vi "NI32LV110ASD8_Dashboard Main 3.vi"() -> ()   [LabVIEW 2011]
uses:
  <vilib>/Rock Robotics/WPI/DriverStation/WPI_DriverStationDigitalData.ctl
  3061 - Robot Code(Bob's)/Dashboard Datatype.ctl
panel:
  in  "Reset":bool
  out "Odometer":dbl
  out "Encoder Odometers":cluster{"Left Encoder":dbl, "Right Encoder":dbl}
  out "Launcher Rate":dbl(slide) scale=0.0..8.0
  out "Image Error Message":string
  in  "Viewer":enum32{"Camera Image", "Kinect Skeleton"}(tab)
  in  "Video Enable":bool
  out "Camera Image":T1(plugin-control)
  out "Buttons 1":cluster{"1":bool, "2":bool, "3":bool}
  out "Kinect 1":cluster{"X":dbl, "Y":dbl, "Z":dbl} {"X" scale=1.0..-1.0; "Y" scale=1.0..-1.0; "Z" scale=1.0..-1.0}
  out "Buttons 2":cluster{"1":bool, "2":bool, "3":bool}
  out "Kinect 2":cluster{"X":dbl, "Y":dbl, "Z":dbl} {"X" scale=1.0..-1.0; "Y" scale=1.0..-1.0; "Z" scale=1.0..-1.0}
  out "Version":string
  out "Skeleton Picture":picture
  out "Players":i8
  out "Robot IP Address":string
  out "Solenoid Output":bool[](array[boolean])
  out "Analog Input":sgl[](array[slide]) scale=0.0..5.0
  out "Relay":cluster{"Forward":bool[], "Reverse":bool[]}
  out "PWM":cluster{u8, u8}[](array[slide]) scale=1.0..255.0
  out "GPIO State":bool[](array[boolean])
  out "GPIO Output Enable":bool[](array[boolean])
  out "8 -- Battery":sgl(graph)
  out "Gyro":cluster{"Robot Gyro":dbl, "Robot Gyro":dbl}(knob) scale=-180.0..180.0
  out "Dashboard Datatype Warning":string
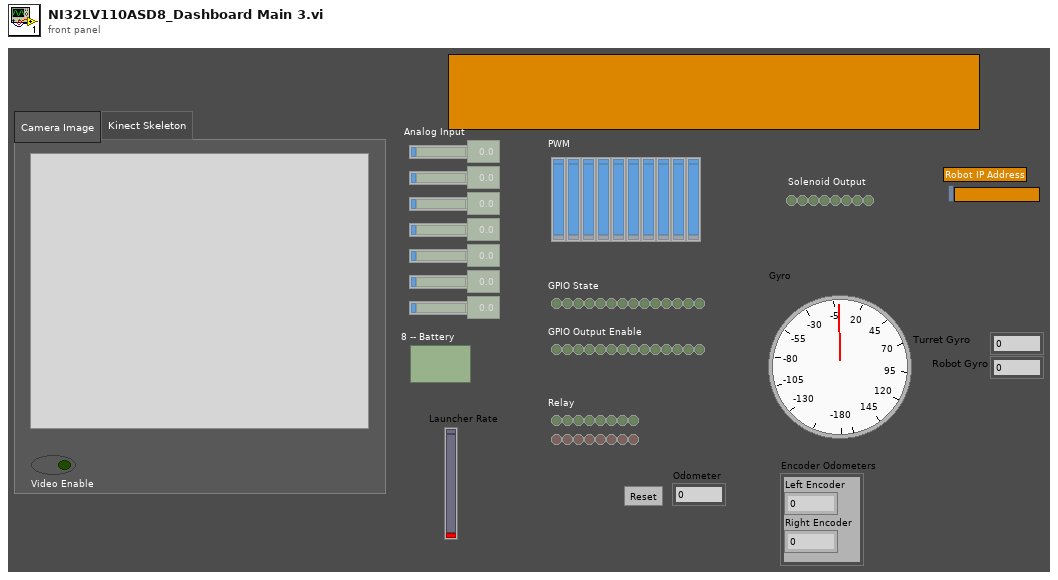
[diagram p1: front panel]
types:
  T1 = typedef "IMAQ Image.ctl" = refnum<image>
  T2 = typedef "Dashboard Datatype.ctl" = cluster{cluster{"AnalogModule[0]":cluster{"Channel[0]":sgl, "Channel[1]":sgl, "Channel[2]":sgl, "Channel[3]":sgl, "Channel[4]":sgl, "Channel[5]":sgl, "Channel[6]":sgl, "Channel[7]":sgl}, "AnalogModule[1]":cluster{"Channel[0]":sgl, "Channel[1]":sgl, "Channel[2]":sgl, "Channel[3]":sgl, "Channel[4]":sgl, "Channel[5]":sgl, "Channel[6]":sgl, "Channel[7]":sgl}}, cluster{"DigitalModule[0]":T3, "DigitalModule[1]":T3}, "Solenoid":u8, "Gyro":dbl, "Wheel Speed":dbl, "Arm Angle":dbl, "Arm Height":dbl, "Rack & Height":string}
  T3 = typedef "WPI_DriverStationDigitalData.ctl" = cluster{"Relay Fwd":u8, "Relay Rev":u8, "GPIO":u16, "GPIO_OE":u16, "PWM":cluster{"PWM[0]":u8, "PWM[1]":u8, "PWM[2]":u8, "PWM[3]":u8, "PWM[4]":u8, "PWM[5]":u8, "PWM[6]":u8, "PWM[7]":u8, "PWM[8]":u8, "PWM[9]":u8}}
  T4 = typedef "Image Type" = u32
  T5 = cluster{"Competition mode":bool, "Robot Link":bool, "Autonomous":bool, "Enabled":bool, "E-Stop":bool}
  T6 = cluster{"AnalogModule[0]":cluster{"Channel[0]":sgl, "Channel[1]":sgl, "Channel[2]":sgl, "Channel[3]":sgl, "Channel[4]":sgl, "Channel[5]":sgl, "Channel[6]":sgl, "Channel[7]":sgl}, "AnalogModule[1]":cluster{"Channel[0]":sgl, "Channel[1]":sgl, "Channel[2]":sgl, "Channel[3]":sgl, "Channel[4]":sgl, "Channel[5]":sgl, "Channel[6]":sgl, "Channel[7]":sgl}}
  T7 = cluster{"DigitalModule[0]":T3, "DigitalModule[1]":T3}
  T8 = cluster{"Channel[0]":sgl, "Channel[1]":sgl, "Channel[2]":sgl, "Channel[3]":sgl, "Channel[4]":sgl, "Channel[5]":sgl, "Channel[6]":sgl, "Channel[7]":sgl}[]
  T9 = cluster{"Channel[0]":sgl, "Channel[1]":sgl, "Channel[2]":sgl, "Channel[3]":sgl, "Channel[4]":sgl, "Channel[5]":sgl, "Channel[6]":sgl, "Channel[7]":sgl}
  T10 = typedef "LVRectTypeDef.ctl" = cluster{"left":i16, "top":i16, "right":i16, "bottom":i16}
  T11 = typedef "SkeletonTrackState.ctl" = enum32{"NotTracked", "PositionOnly", "Tracked"}
  T12 = cluster{"TrackingState":u8[], "Position":cluster{"x":sgl, "y":sgl, "z":sgl}, cluster{"x":sgl, "y":sgl, "z":sgl, sgl}[], "TrackState":T11}
  T13 = cluster{cluster{"ScaledToPercentRange":dbl, "ScaledToPercentRange":dbl, "ScaledToPercentRange":dbl}, cluster{bool, bool, bool}}[]
  T14 = typedef "LVBoundsTypeDef.ctl" = cluster{"Width":u32, "Height":u32}
  T15 = cluster{cluster{"ScaledToPercentRange":dbl, "ScaledToPercentRange":dbl, "ScaledToPercentRange":dbl}, cluster{bool, bool, bool}}
  T16 = cluster{"ScaledToPercentRange":dbl, "ScaledToPercentRange":dbl, "ScaledToPercentRange":dbl}
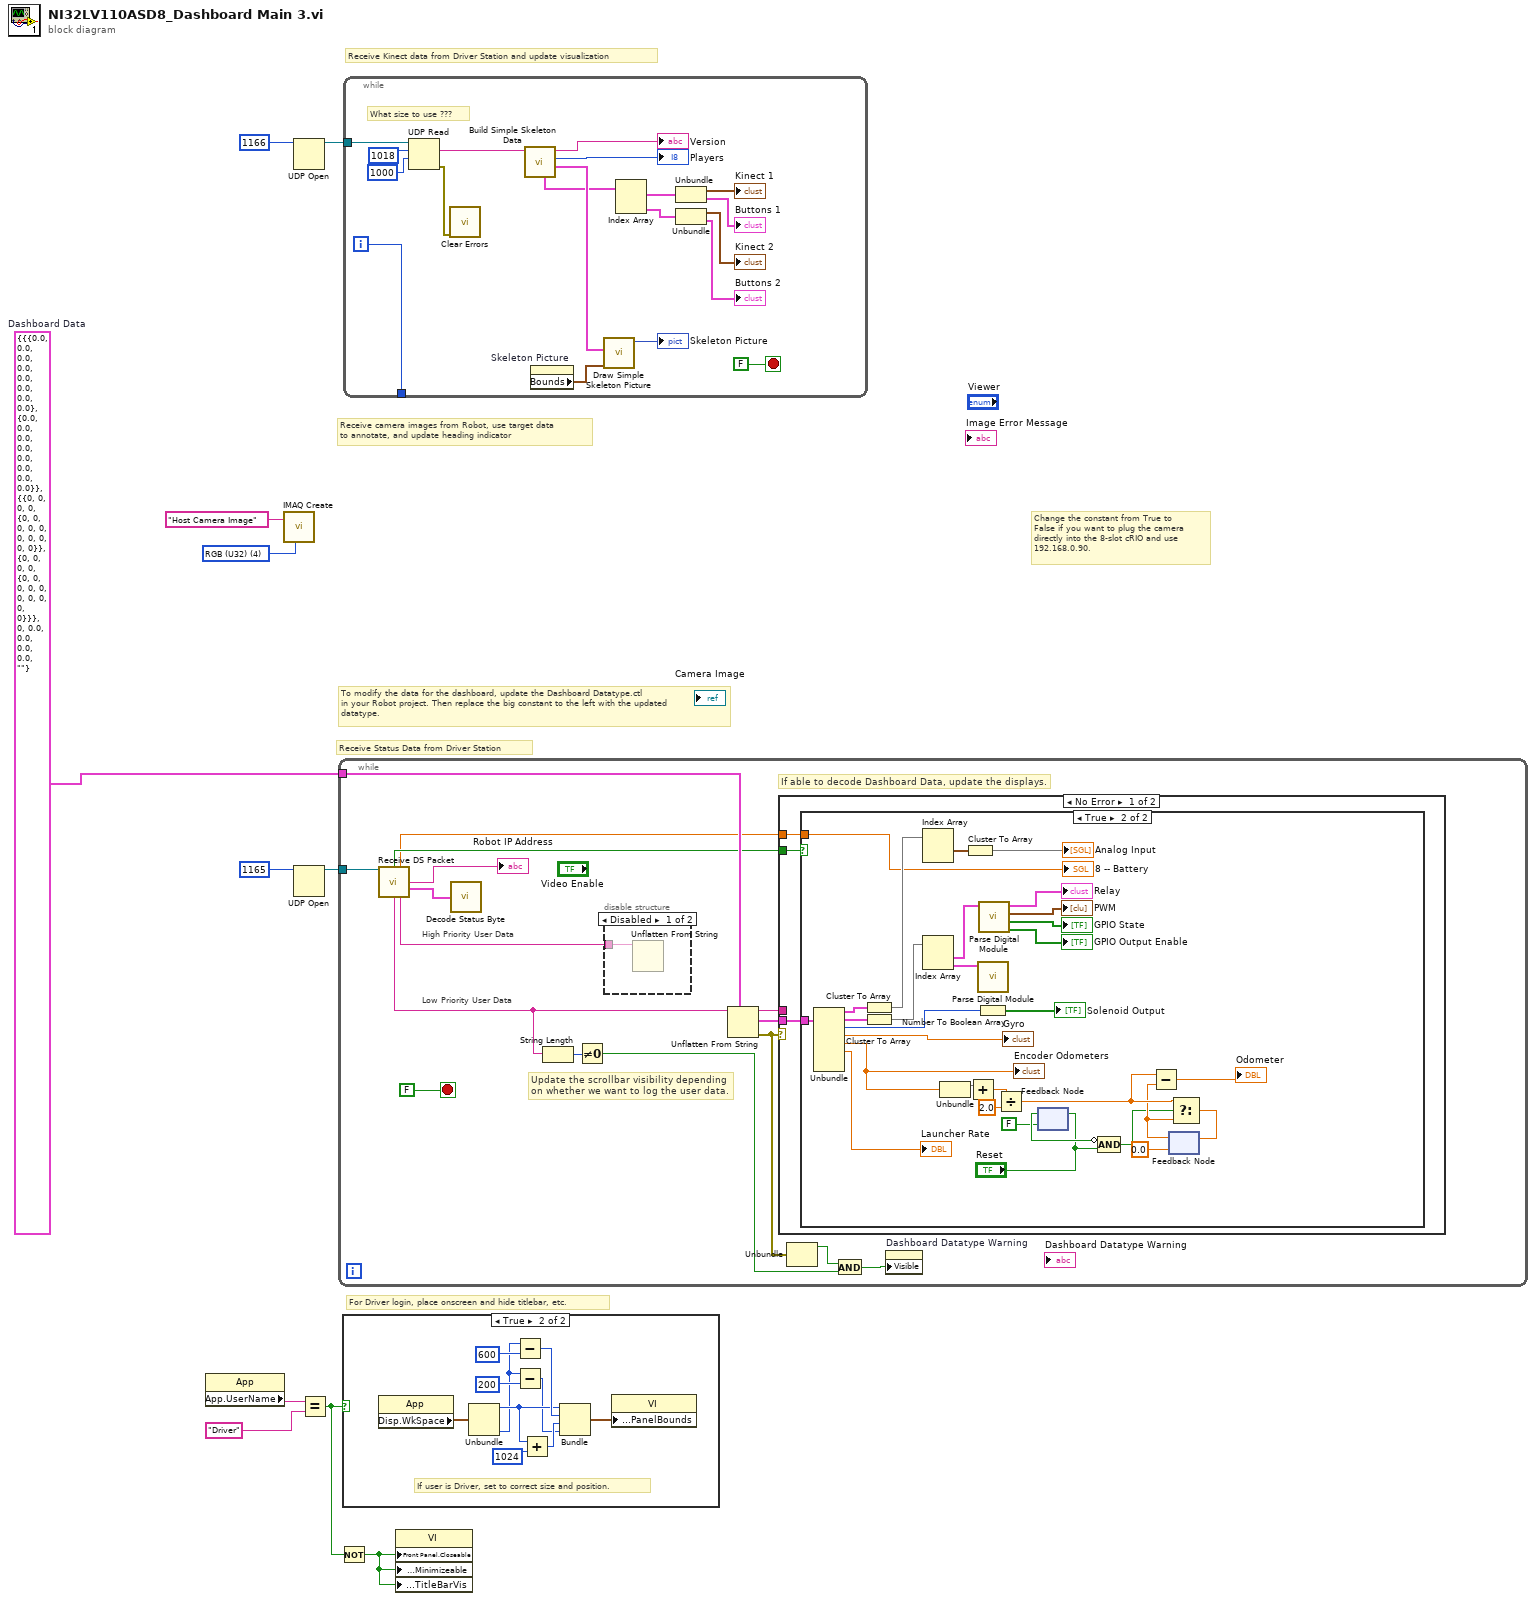
[diagram p0: block diagram]
diagram:
  w1 = T2 {{"AnalogModule[0]"={"Channel[0]"=0.0, "Channel[1]"=0.0, "Channel[2]"=0.0, "Channel[3]"=0.0, "Channel[4]"=0.0, "Channel[5]"=0.0, "Channel[6]"=0.0, "Channel[7]"=0.0}, "AnalogModule[1]"={"Channel[0]"=0.0, "Channel[1]"=0.0, "Channel[2]"=0.0, "Channel[3]"=0.0, "Channel[4]"=0.0, "Channel[5]"=0.0, "Channel[6]"=0.0, "Channel[7]"=0.0}}, {"DigitalModule[0]"={"Relay Fwd"=0, "Relay Rev"=0, "GPIO"=0, "GPIO_OE"=0, "PWM"={"PWM[0]"=0, "PWM[1]"=0, "PWM[2]"=0, "PWM[3]"=0, "PWM[4]"=0, "PWM[5]"=0, "PWM[6]"=0, "PWM[7]"=0, "PWM[8]"=0, "PWM[9]"=0}}, "DigitalModule[1]"={"Relay Fwd"=0, "Relay Rev"=0, "GPIO"=0, "GPIO_OE"=0, "PWM"={"PWM[0]"=0, "PWM[1]"=0, "PWM[2]"=0, "PWM[3]"=0, "PWM[4]"=0, "PWM[5]"=0, "PWM[6]"=0, "PWM[7]"=0, "PWM[8]"=0, "PWM[9]"=0}}}, "Solenoid"=0, "Gyro"=0.0, "Wheel Speed"=0.0, "Arm Angle"=0.0, "Arm Height"=0.0, "Rack & Height"=""}  # Dashboard Data
  w9 = T4 4 items=["Grayscale (U8)", "Grayscale (I16)", "Grayscale (SGL)", "Complex (CSG)", "RGB (U32)", "HSL (U32)", "RGB (U64)"] ("Image Type")
  # "Change the constant from True to\nFalse if you want to plug the camera\ndirectly into the 8-slot cRIO and use\n192.168.0.90."
  # "Receive Kinect data from Driver Station and update visualization"
  # "For Driver login, place onscreen and hide titlebar, etc."
  # "To modify the data for the dashboard, update the Dashboard Datatype.ctl\nin your Robot project. Then replace the big constant to the left with the updated\ndatatype."
  # "Receive Status Data from Driver Station"
  # "Receive camera images from Robot, use target data\nto annotate, and update heading indicator"
  n1 = property class="App"() -> ("App.UserName"=w6:string)  [unwired: 2 in, 2 out]
  n2 = call "IMAQ Create"("Image Name"="Host Camera Image", "Image Type"=w9) -> ()  [unwired: 2 in, 3 out]
  n3 = UDP Open(11:u16 1166 ("port")) -> (port=w2:refnum<k16>)  [unwired: 2 in, 4 out]
  n4 = UDP Open(11:u16 1165 ("port")) -> (port=w10:refnum<k16>)  [unwired: 2 in, 4 out]
  n5 = Equal?(x=w6, y="Driver") -> (x = y?=w5:bool)
  n6 = while {
    tunnel: w10 -> [w25]
    tunnel: w1 -> [w24]
    stop <- FALSE stop-if-true
    # "High Priority User Data"
    # "Low Priority User Data"
    # "Update the scrollbar visibility depending\non whether we want to log the user data."
    # "If able to decode Dashboard Data, update the displays."
    n7 = call "Receive DS Packet.vi"("Recv Socket"=w25) -> ("New Dashboard Data"=w21:bool, "Battery"=w12:sgl, "Robot IP Address"=→"Robot IP Address":string, "Status"=w26:T5, "Low Priority User Data"=w14:string, "High Priority User Data"=w13:string)  [unwired: 1 in, 8 out]
    n8 = call "Decode Status Byte.vi"("Status Byte"=w26) -> ()  [unwired: 2 out]
    n9 = String Length(string=w14) -> (length=w16:i32)
    n10 = Not Equal To 0?(x=w16) -> (x != 0?=w19:bool)
    n11 = disable-structure shown="Disabled" {
      disable-tunnel: w13 -> [w28 _]
      frame Disabled {
        n12 = Unflatten From String(binary string=w28) -> ()  [unwired: 2 in, 5 out]
      }
      frame Enabled {
      }
    }
    n13 = Unflatten From String(type=w24, binary string=w14) -> (rest of the binary string=w17:string, value=w23:T2, error out=w22:errorcluster)  [unwired: 1 in, 2 out]
    n14 = case shown="No Error" w22 {
      tunnel: w23 -> [w31 _]
      tunnel: w21 -> [w30 _]
      tunnel: w17 -> [_ _]
      tunnel: w12 -> [w29 _]
      frame No Error {
        n15 = case shown="True" w30 {
          tunnel: w31 -> [_ w54]
          tunnel: w29 -> [_ w48]
          frame False {
            # "Don't update if the robot hasn't sent new data"
          }
          frame True {
            n16 = Unbundle(w54) -> (w51:T6, w52:T7, "Solenoid"=w53:u8, "Gyro"=→"Gyro":dbl, "Wheel Speed"=w45:dbl, "Arm Angle"=→"Launcher Rate":dbl)  [unwired: 2 out]
            "Encoder Odometers" <- w45
            n17 = Cluster To Array(cluster=w51) -> (array=w62:T8)
            n18 = Cluster To Array(cluster=w52) -> (array=w61:T3[])
            n19 = Index Array(array=w62) -> (element #1=w49:T9)  [unwired: 2 in, 1 out]
            n20 = Index Array(array=w61) -> (element #1=w60:T3, element #2=w55:T3)  [unwired: 2 in]
            n21 = Unbundle(w45) -> (w43, w44)
            n22 = Cluster To Array(cluster=w49) -> (array=→"Analog Input":sgl[])
            n23 = Add(x=w43, y=w44) -> (x+y=w42:dbl)
            n24 = call "Parse Digital Module.vi"("DigitalModule"=w55) -> ()  [unwired: 11 out]
            n25 = Number To Boolean Array(number=w53) -> (Boolean array=→"Solenoid Output":bool[])
            n26 = call "Parse Digital Module.vi"("DigitalModule"=w60) -> ("GPIO Output Enable"=→"GPIO Output Enable":bool[], "GPIO State"=→"GPIO State":bool[], "PWM"=→"PWM":cluster{u8, u8}[], "Relay"=→"Relay":cluster{"Forward":bool[], "Reverse":bool[]})  [unwired: 7 out]
            n27 = Divide(x=w42, y=2.0) -> (x/y=w39:dbl)
            n28 = feedback #1(FALSE ("Reset")) -> (w35:bool)
            n29 = feedback-in #1("Reset") -> ()
            n30 = Compound Arithmetic op=AND(invert w35, "Reset") -> (w33:bool)
            n31 = feedback #2(0.0) -> (w38:dbl)
            n32 = Subtract(x=w39, y=w38) -> (x-y=→"Odometer":dbl)
            n33 = Select(t=w39, s=w33, f=w38) -> (s? t:f=w37:dbl)
            n34 = feedback-in #2(w37) -> ()
            "8 -- Battery" <- w48
          }
        }
      }
      frame Error {
        # "Your datatypes don't match. The Dashboard Datatype.ctl in your Robot project\nand the big constant to the left of the loop need to match."
      }
    }
    n35 = Unbundle(w22) -> ("status"=w18:bool)  [unwired: 2 out]
    n36 = And(x=w18, y=w19) -> (x .and. y?=w20:bool)
    n37 = property on="Dashboard Datatype Warning" class="Str"("Visible"=w20) -> ()  [unwired: 2 in, 2 out]
  }
  n38 = Not(x=w5) -> (.not. x?=w4:bool)
  n39 = case shown="True" w5 {
    frame False {
    }
    frame True {
      # "If user is Driver, set to correct size and position."
      n40 = property class="App"() -> ("Disp.WkSpace"=w73:T10)  [unwired: 2 in, 2 out]
      n41 = Unbundle(w73) -> ("left"=w68:i16, "bottom"=w64:i16)  [unwired: 2 out]
      n42 = Subtract(x=w64, y=600) -> (x-y=w70:i32)
      n43 = Subtract(x=w64, y=200) -> (x-y=w65:i32)
      n44 = Add(x=w68, y=1024) -> (x+y=w69:i32)
      n45 = Bundle("left"=w68, w70, w69, w65) -> (w72:cluster{"left":i16, i32, i32, i32})  [unwired: 1 out]
      n46 = property class="VI"("Front Panel.PanelBounds"=w72) -> ()  [unwired: 2 in, 2 out]
    }
  }
  n47 = while {
    tunnel: w2 -> [w90]
    tunnel: [w74] -> _
    i -> [w74]
    stop <- FALSE stop-if-true
    # "What size to use ???"
    n48 = UDP Read(connection ID=w90, max size (548)=1018 ("bytes to read"), timeout ms (25000)=1000) -> (data out=w84:string, error out=w82:errorcluster)  [unwired: 1 in, 3 out]
    n49 = call <vilib>:"Clear Errors.vi"("error in (no error)"=w82) -> ()  [unwired: 6 in, 1 out]
    n50 = call "Build Simple Skeleton Data.vi"("data out"=w84) -> ("Skeleton Data"=w85:T12, "NumPlayers"=→"Players":i8, "Version String"=→"Version":string, "Simple Joystick Info"=w81:T13)  [unwired: 6 in, 1 out]
    n51 = property on="Skeleton Picture" class="Pict"() -> ("Bounds"=w86:T14)  [unwired: 2 in, 2 out]
    n52 = call "Draw Simple Skeleton Picture.vi"("Bounds"=w86, "Simple Skeleton"=w85) -> ("new picture out"=→"Skeleton Picture":picture)  [unwired: 9 in]
    n53 = Index Array(array=w81) -> (element #1=w80:T15, element #2=w79:T15)  [unwired: 2 in]
    n54 = Unbundle(w80) -> (→"Kinect 1":T16, →"Buttons 1":cluster{bool, bool, bool})
    n55 = Unbundle(w79) -> (→"Kinect 2":T16, →"Buttons 2":cluster{bool, bool, bool})
  }
  n56 = property class="VI"("Front Panel.Closeable"=w4, "Front Panel.Minimizeable"=w4, "Front Panel.TitleBarVis"=w4) -> ()  [unwired: 2 in, 2 out]
